vi "Get FP Items Refs Map.vi"(8 "error in (no error)":errorcluster, 10 "ID":string, 11 "uService List in":refnum<class "uService List.lvclass">) -> (0 "error out":errorcluster, 2 "FP Items Refs Map":map{string, refnum<vi>}(c390), 3 "uService List out":refnum<class "uService List.lvclass">)   [LabVIEW 2026, in "TALOS.lvlib" / "Classes.lvlib" / "uService List.lvclass"]
uses:
  uService List.lvclass
  uService List.lvclass/uService List.ctl
  Ancestor/Ancestor/Ancestor.lvclass/Ancestor.ctl
  FGV/Error Memory/Get Error Description.vi
  Support VIs/Get PC name.vi
  Ancestor/Ancestor/Read ID.vi
  Support VIs/Get Class Name.vi
  <vilib>/Utility/error.llb/Clear Errors.vi
  FGV/Error Memory/Error Memory Core.vi
  <vilib>/AdvancedString/Delimited String to 1D String Array.vi
  <vilib>/AdvancedString/Delimited String to 1D String Array (string).vi
  Support VIs/Circus Root Path.vi
  FGV/Error Memory/Error Crt Lvl checker.vi
  FGV/Error Memory/Error Memory Core.vi/40c8088d-b597-4017-91af-faa98e00292e.vi
  FGV/Error Memory/Error Memory Core.vi/d4a3ab98-063c-4e44-b43d-fbdcfe6c2be2.vi
  Support VIs/Global Memory.vi
  <vilib>/Utility/LVClass/Get LV Class Name.vi
  Support VIs/Is in Packed Library.vi
  Support VIs/TALOS Root path.vi
  Support VIs/Read CSV worksheet.vi
  Support VIs/Global Constants.vi
  <vilib>/Utility/error.llb/General Error Handler.vi
  Ancestor/Ancestor/Ancestor.lvclass
  <vilib>/Comparison/Equal/Equal Functor/Equal Functor.lvclass
  TALOS.lvlib
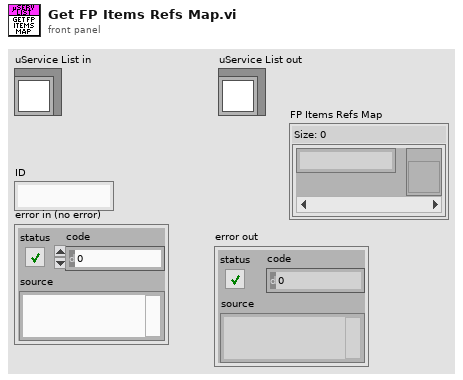
[diagram p1: front panel]
types:
  T1 = typedef "TALOS.lvlib/Classes.lvlib/uService List.lvclass/uService Properties.ctl" = cluster{"uService Queue":refnum<class "Message Enqueuer.lvclass">, "Last Pat":timestamp, "Online":bool, "Vi Ref":refnum<vi>, "Class name":string, "GUI":bool, "FP Items Refs Map":map{string, refnum<vi>}, "Remote GUI":bool, "Remote Window":refnum<vi>}
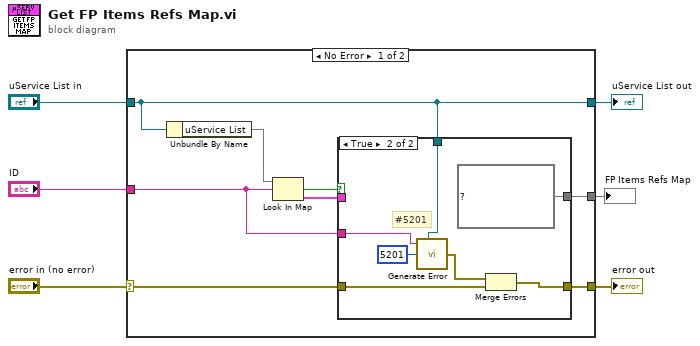
[diagram p0: block diagram]
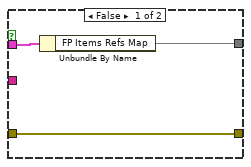
[diagram p2: hidden frame]
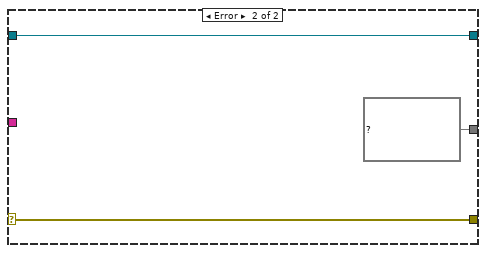
[diagram p3: hidden frame]
diagram:
  n1 = case shown="No Error" "error in (no error)" {
    selector: "error in (no error)" -> [w13 w27]
    tunnel: "uService List in" -> [w7 w26]
    tunnel: [w11 w27] -> w4
    tunnel: [w7 w26] -> w3
    tunnel: "ID" -> [w8 _]
    tunnel: [w9 map{string, refnum<vi>} {} ("FP Items Refs Map")] -> w1
    frame No Error {
      n2 = Unbundle By Name(w7) -> ("uService List"=w14:map{string, T1})
      n3 = Look In Map(map=w14, key=w8) -> (key not found?=w12:bool, value=w10:T1)  [unwired: 1 in]
      n4 = case shown="True" w12 {
        tunnel: w13 -> [w17 w22]
        tunnel: [w17 w21] -> w11
        tunnel: w10 -> [w16 _]
        tunnel: [w15 map{string, refnum<vi>} {} ("FP Items Refs Map")] -> w9
        tunnel: w8 -> [_ w19]
        tunnel: w7 -> [_ w18]
        frame False {
          n5 = Unbundle By Name(w16) -> ("FP Items Refs Map"=w15:map{string, refnum<vi>})
        }
        frame True {
          # "#5201"
          n6 = call "Generate Error.vi"("Optional String"=w19, "Class"=w18, "Error Code"=5201) -> ("error out"=w23:errorcluster)  [unwired: 4 in]
          n7 = Merge Errors(w23, w22) -> (w21:errorcluster)
        }
      }
    }
    frame Error {
    }
  }
  "error out" <- w4
  "uService List out" <- w3
  "FP Items Refs Map" <- w1
